vi "FTW-Actor-Publish.vi"(0 "FTW Actor Instance":refnum<class "FTW-Actor-Instance.lvclass">, 5 "Message":string, 7 "Topic":string, 9 "Timeout":i32 format="%dmsec", 11 "error in":errorcluster) -> (4 "FTW Actor Instance out":refnum<class "FTW-Actor-Instance.lvclass">, 6 "Timed out?":bool, 15 "error out":errorcluster)   [LabVIEW 2013, in "FTW-Actor-Instance.lvclass"]
uses:
  FTW-Actor-Instance.lvclass
  FTW-Actor-Instance.lvclass/FTW-Actor-Instance.ctl
  socket/FTW-Socket.lvclass
panel:
  # "Inputs"
  # "Outputs"
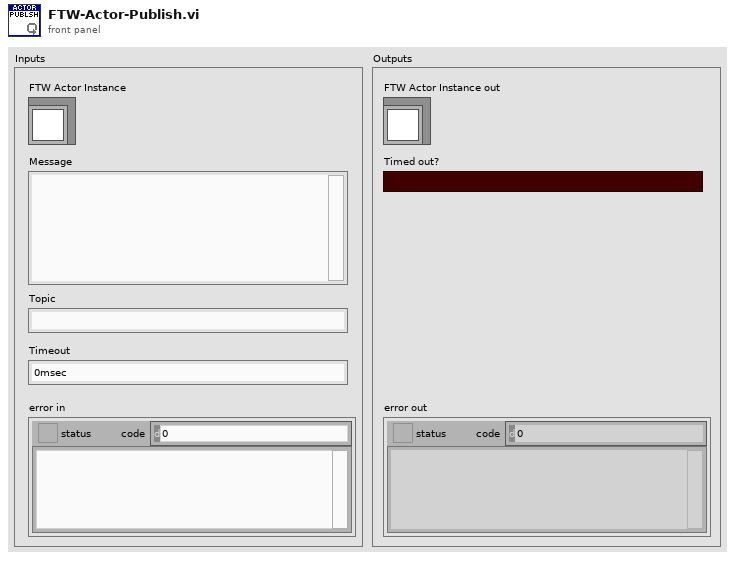
[diagram p1: front panel]
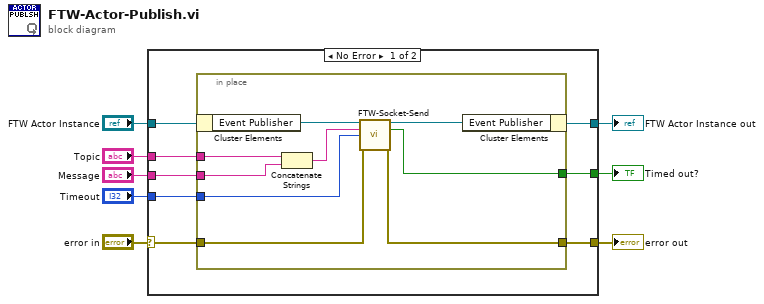
[diagram p0: block diagram]
diagram:
  n1 = case shown="No Error" "error in" {
    selector: "error in" -> [w15 w27]
    tunnel: [w13 w27] -> w7
    tunnel: "FTW Actor Instance" -> [w16 w26]
    tunnel: [w14 w26] -> w5
    tunnel: "Topic" -> [w12 _]
    tunnel: "Message" -> [w11 _]
    tunnel: "Timeout" -> [w10 _]
    tunnel: [w9 _] -> w1
    frame No Error {
      n2 = in-place {
        in-place-border: w15 -> [w25]
        in-place-border: [w24] -> w13
        in-place-border: w12 -> [w20]
        in-place-border: w11 -> [w19]
        in-place-border: w10 -> [w17]
        in-place-border: [w21] -> w9
        n3 = in-place-cluster #1(w16) -> ("Event Publisher"=w23:refnum<class "FTW-Socket.lvclass">)
        n4 = Concatenate Strings(w20, w19) -> (w18:string)
        n5 = call "FTW-Socket-Send.vi"("FTW Socket"=w23, "Message"=w18, "Send Timeout"=w17, "error in"=w25) -> ("FTW Socket out"=w22:refnum<class "FTW-Socket.lvclass">, "Timed out?"=w21:bool, "error out"=w24:errorcluster)  [unwired: 9 in]
        n6 = in-place-cluster #1("Event Publisher"=w22) -> (w14:refnum<class "FTW-Actor-Instance.lvclass">)
      }
    }
    frame Error {
    }
  }
  "error out" <- w7
  "FTW Actor Instance out" <- w5
  "Timed out?" <- w1
